vi "Scan_Rate_Mon.vi"() -> (0 "Heart rate(s)":dbl format="%#_6p", 1 "Execute rate(Hz)":dbl format="%#_6p")   [LabVIEW 2021]
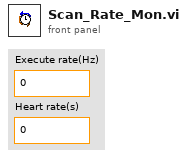
[diagram p1: front panel]
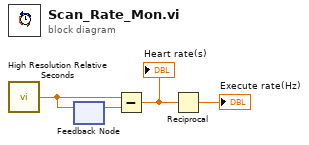
[diagram p0: block diagram]
diagram:
  n1 = call <vilib>:"High Resolution Relative Seconds.vi"() -> ("relative seconds"=w3:dbl)
  n2 = feedback #1() -> (w4:dbl)  [unwired: 1 in]
  n3 = feedback-in #1(w3) -> ()
  n4 = Subtract(x=w3, y=w4) -> (x-y=w2:dbl)
  "Heart rate(s)" <- w2
  n5 = Reciprocal(x=w2) -> (1/x=→"Execute rate(Hz)":dbl)
